vi "Config Program.vi"(8 "error in (no error)":errorcluster, 11 "Prog in":T1) -> (0 "error out":errorcluster, 3 "Prog out":T1)   [LabVIEW 2014, in "SeqLoop.lvlib"]
doc: "Configura un Programa que contiene la secuencias de autocero, ciclo y especiales."
uses:
  SeqLoop.lvlib
  TypeDefs/Program.ctl
  TypeDefs/Sequence.ctl
  TypeDefs/STEP.ctl
  TypeDefs/LogicParsedExpression.ctl
  Mimico Display/TypeDefs/Mimic Data.ctl
  Mimico Display/TypeDefs/BG Image.ctl
  Mimico Display/TypeDefs/mObject.ctl
  Mimico Display/Mimico Display.lvlib
panel:
  in  "Total Meds. Aux.:":i32
  in  "Total Meds.:":i32
  in  "Save":bool
  in  "Close":bool
  in  "Config AutoZero":bool
  in  "Diseño":string
  in  "Autor":string
  in  "Nombre Programa":string
  in  "Descripción":string
  in  "Pieza":i32
  in  "Operación":i32
  in  "Config Measurement":bool
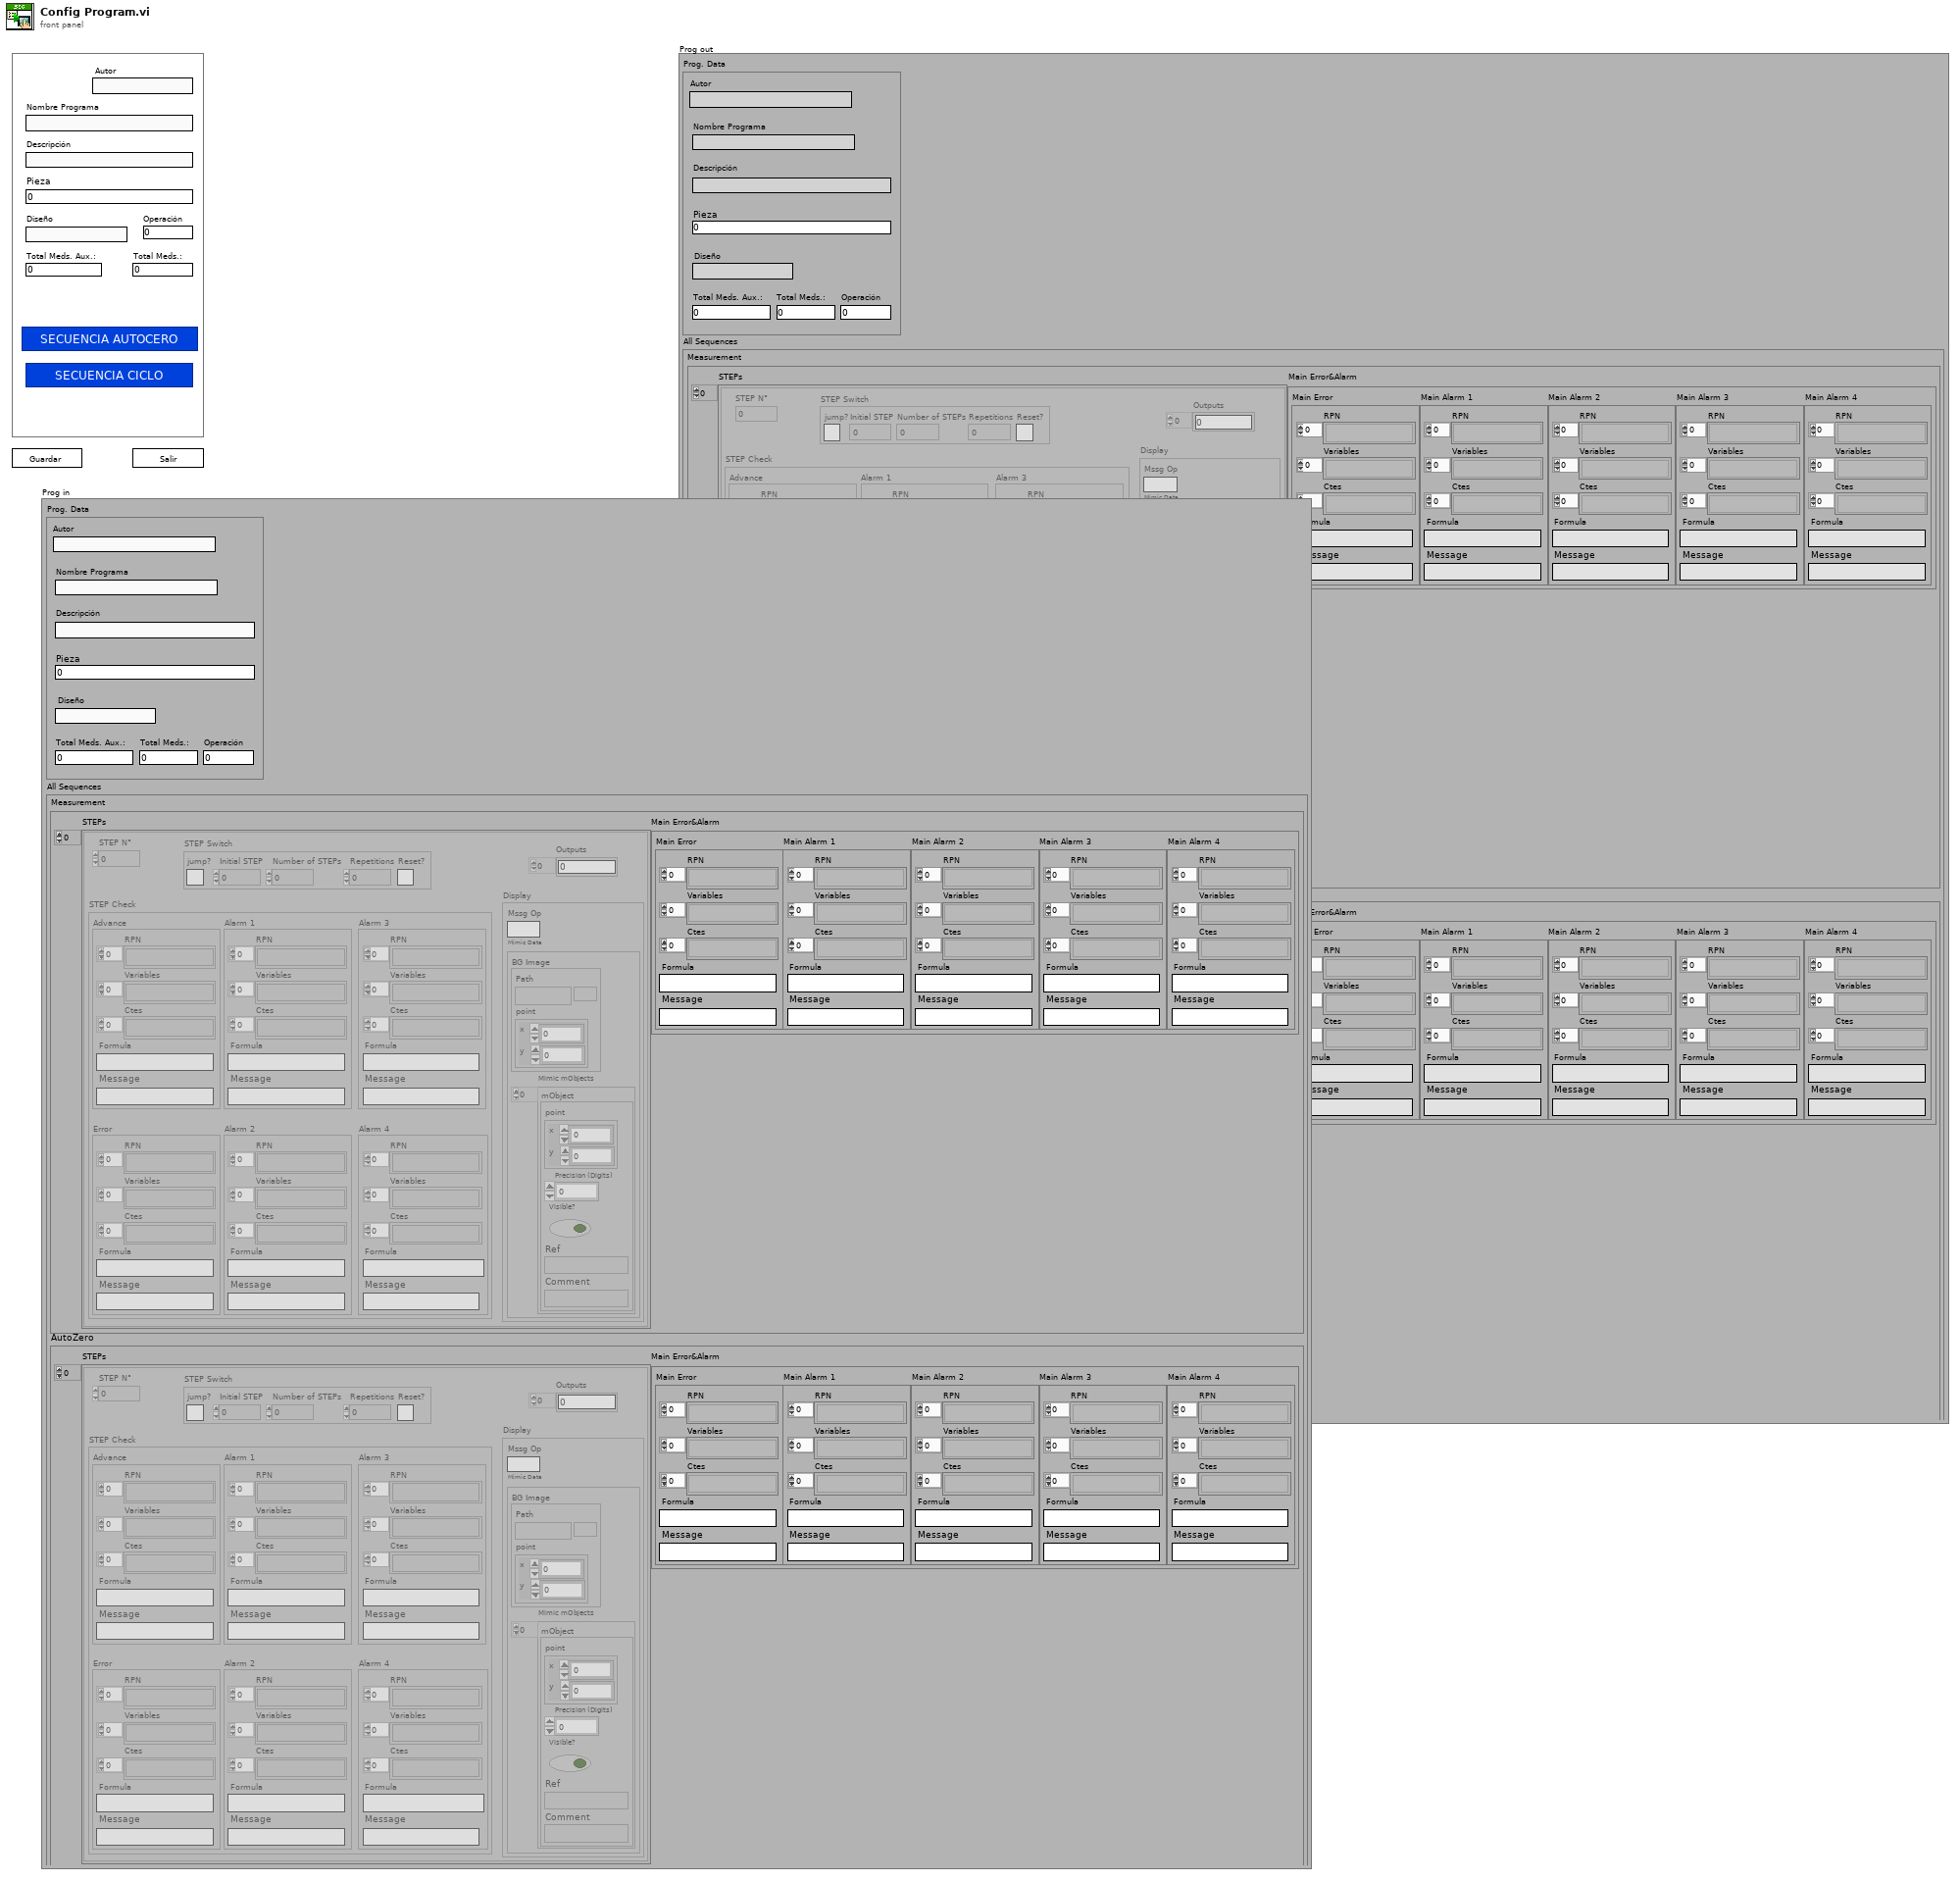
[diagram p1: front panel]
types:
  T1 = typedef "SeqLoop.lvlib/Program.ctl" = cluster{"Prog. Data":cluster{"Operación":i32, "Pieza":i32, "Descripción":string, "Nombre Programa":string, "Autor":string, "Diseño":string, "Total Meds.:":i32, "Total Meds. Aux.:":i32}, "All Sequences":cluster{"Measurement":T2, "AutoZero":T2}}
  T2 = typedef "SeqLoop.lvlib/Sequence.ctl" = cluster{"STEPs":T3[], "Main Error&Alarm":cluster{"Main Error":T4, "Main Alarm 1":T4, "Main Alarm 2":T4, "Main Alarm 3":T4, "Main Alarm 4":T4}}
  T3 = typedef "SeqLoop.lvlib/STEP.ctl" = cluster{"STEP N°":u32, "STEP Switch":cluster{"jump?":bool, "Initial STEP":u32, "Number of STEPs":u32, "Repetitions":u32, "Reset?":bool}, "Outputs":i32[], "STEP Check":cluster{"Advance":T4, "Error ":T4, "Alarm 1":T4, "Alarm 2":T4, "Alarm 3":T4, "Alarm 4":T4}, "Display":cluster{"Mssg Op":string, "Mimic Data":T5}}
  T4 = typedef "SeqLoop.lvlib/LogicParsedExpression.ctl" = cluster{"RPN ":string[], "Variables":string[], "Ctes":string[], "Formula":string, "Message":string}
  T5 = typedef "SeqLoop.lvlib/Mimico Display.lvlib/Mimic Data.ctl" = cluster{"BG Image":T6, "Mimic mObjects":T7[]}
  T6 = typedef "SeqLoop.lvlib/Mimico Display.lvlib/BG Image.ctl" = cluster{"Path":path, "point":cluster{"x":i16, "y":i16}}
  T7 = typedef "SeqLoop.lvlib/Mimico Display.lvlib/mObject.ctl" = cluster{"point":cluster{"x":i16, "y":i16}, "Precision (Digits)":i32, "Visible?":bool, "Ref":string, "Comment":string}
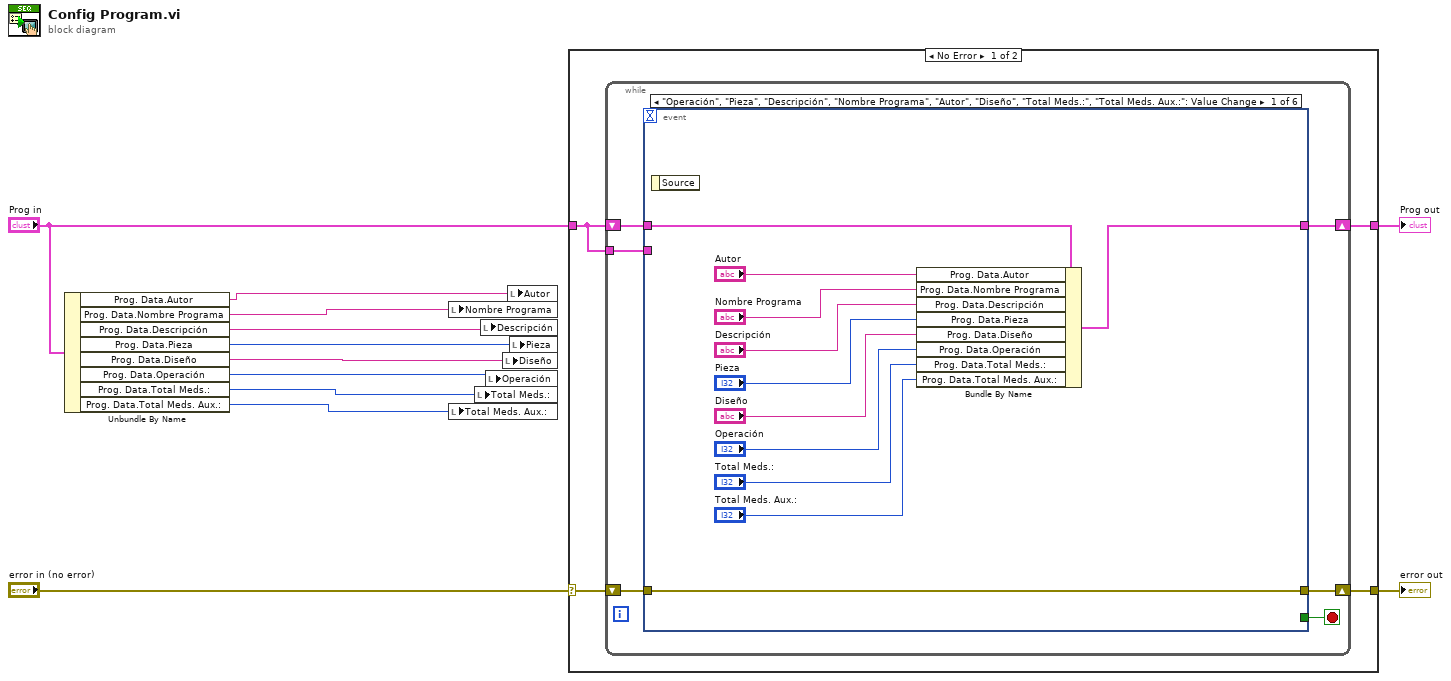
[diagram p0: block diagram]
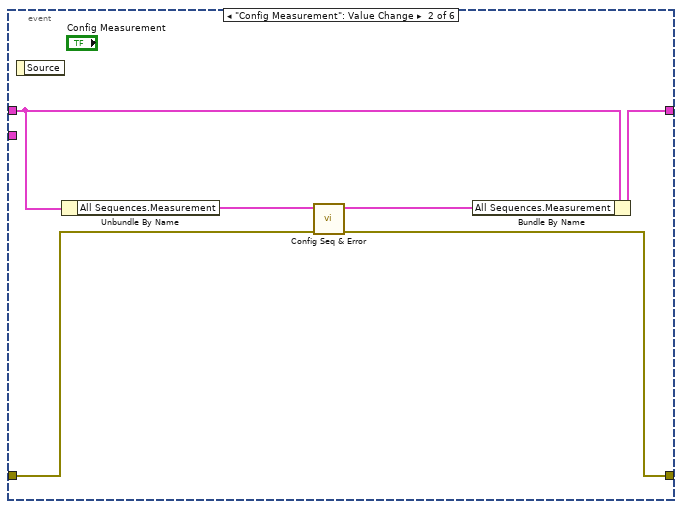
[diagram p2: hidden frame]
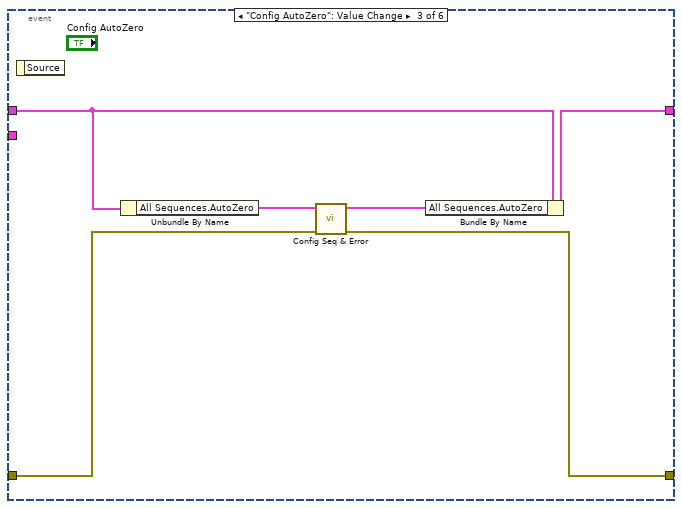
[diagram p3: hidden frame]
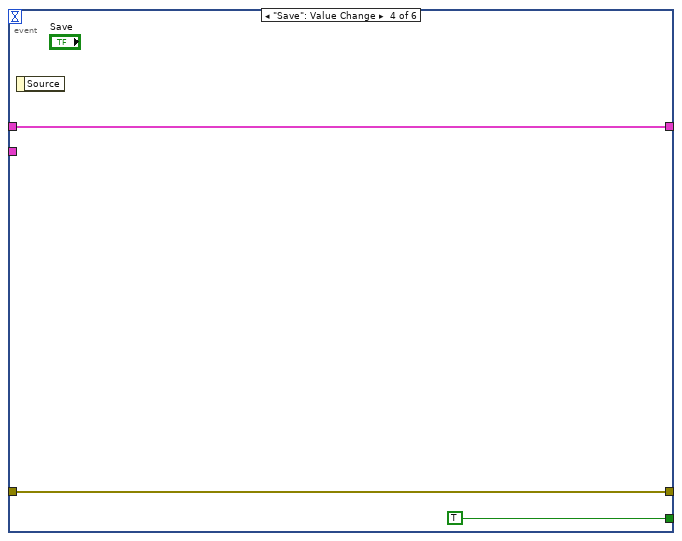
[diagram p4: hidden frame]
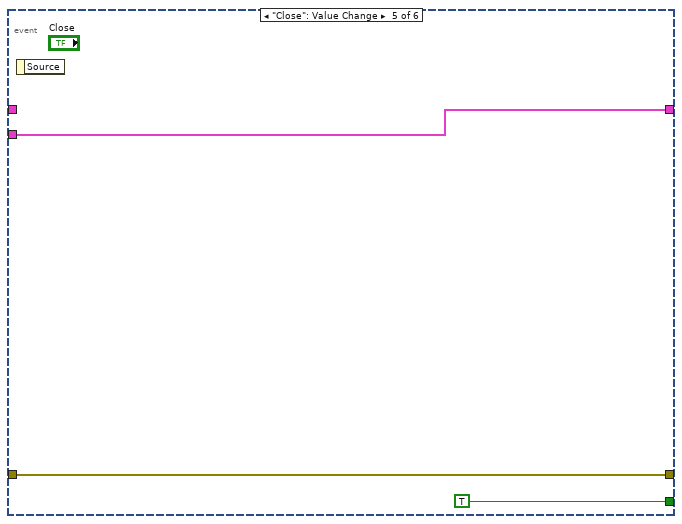
[diagram p5: hidden frame]
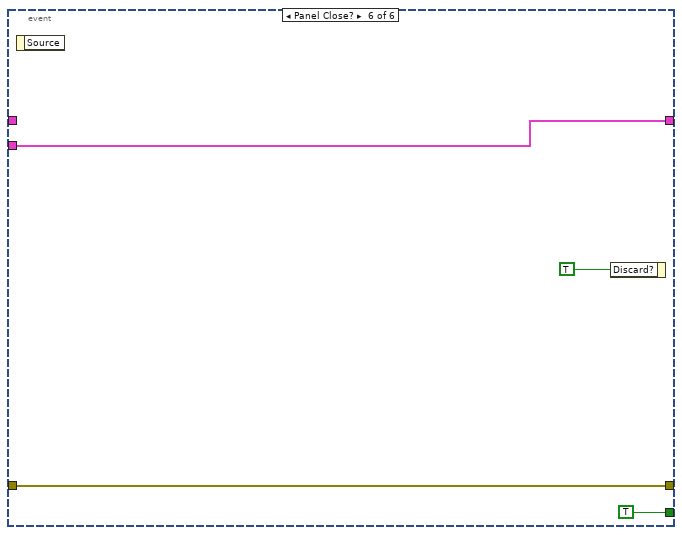
[diagram p6: hidden frame]
diagram:
  n1 = Unbundle By Name("Prog in") -> ("Prog. Data.Autor"=w1:string, "Prog. Data.Nombre Programa"=w8:string, "Prog. Data.Descripción"=w7:string, "Prog. Data.Pieza"=w6:i32, "Prog. Data.Diseño"=w5:string, "Prog. Data.Operación"=w4:i32, "Prog. Data.Total Meds.:"=w3:i32, "Prog. Data.Total Meds. Aux.:"=w2:i32)
  n2 = local write "Nombre Programa"(w8) -> ()
  n3 = local write "Total Meds. Aux.:"(w2) -> ()
  n4 = local write "Total Meds.:"(w3) -> ()
  n5 = local write "Descripción"(w7) -> ()
  n6 = local write "Operación"(w4) -> ()
  n7 = local write "Diseño"(w5) -> ()
  n8 = local write "Autor"(w1) -> ()
  n9 = local write "Pieza"(w6) -> ()
  n10 = case shown="No Error" "error in (no error)" {
    selector: "error in (no error)" -> [w16 w57]
    tunnel: [w15 w57] -> w11
    tunnel: "Prog in" -> [w13 w56]
    tunnel: [w14 w56] -> w10
    frame No Error {
      n11 = while {
        shift-right: [w21] -> w15
        shift-left: w16 -> [w22]
        shift-right: [w19] -> w14
        shift-left: w13 -> [w20]
        tunnel: w13 -> [w17]
        stop <- w18 stop-if-true
        n12 = event shown="[0] \"Operación\", \"Pieza\", \"Descripción\", \"Nombre Programa\", \"Autor\", \"Diseño\", \"Total Meds.:\", \"Total Meds. Aux.:\": Value Change" {
          selector: _ -> [_ _ _ _ _ _]
          dyn-events: _ -> [_ _ _ _ _ _]
          timeout: _ -> [_ _ _ _ _ _]
          tunnel: w22 -> [w33 w35 w40 w47 w49 w54]
          tunnel: [w33 w34 w41 w47 w49 w54] -> w21
          tunnel: w20 -> [w32 w39 w45 w46 _ _]
          tunnel: [w31 w38 w44 w46 w51 w52] -> w19
          tunnel: [_ _ _ TRUE TRUE TRUE] -> w18
          tunnel: w17 -> [_ _ _ _ w51 w52]
          event "Operación", "Pieza", "Descripción", "Nombre Programa", "Autor", "Diseño", "Total Meds.:", "Total Meds. Aux.:": Value Change {
            n13 = event-data() -> ()  [unwired: 1 in, 1 out]
            n14 = Bundle By Name(cluster=w32, "Prog. Data.Autor"="Autor", "Prog. Data.Nombre Programa"="Nombre Programa", "Prog. Data.Descripción"="Descripción", "Prog. Data.Pieza"="Pieza", "Prog. Data.Diseño"="Diseño", "Prog. Data.Operación"="Operación", "Prog. Data.Total Meds.:"="Total Meds.:", "Prog. Data.Total Meds. Aux.:"="Total Meds. Aux.:") -> (w31:T1)
          }
          event "Config Measurement": Value Change {
            n15 = event-data() -> ()  [unwired: 1 in, 1 out]
            n16 = Unbundle By Name(w39) -> ("All Sequences.Measurement"=w36:T2)
            n17 = call "Config Seq & Error.vi"("error in (no error)"=w35, "Sequences"=w36) -> ("error out"=w34:errorcluster, "Sequences"=w37:T2)  [unwired: 8 in]
            n18 = Bundle By Name(cluster=w39, "All Sequences.Measurement"=w37) -> (w38:T1)
          }
          event "Config AutoZero": Value Change {
            n19 = event-data() -> ()  [unwired: 1 in, 1 out]
            n20 = Unbundle By Name(w45) -> ("All Sequences.AutoZero"=w43:T2)
            n21 = call "Config Seq & Error.vi"("error in (no error)"=w40, "Sequences"=w43) -> ("error out"=w41:errorcluster, "Sequences"=w42:T2)  [unwired: 8 in]
            n22 = Bundle By Name(cluster=w45, "All Sequences.AutoZero"=w42) -> (w44:T1)
          }
          event "Save": Value Change {
            n23 = event-data() -> ()  [unwired: 1 in, 1 out]
          }
          event "Close": Value Change {
            n24 = event-data() -> ()  [unwired: 1 in, 1 out]
          }
          event Panel Close? {
            n25 = event-data() -> ()  [unwired: 1 in, 1 out]
            n26 = event-data("Discard?"=TRUE) -> ()  [unwired: 1 in, 1 out]
          }
        }
      }
    }
    frame Error {
    }
  }
  "error out" <- w11
  "Prog out" <- w10
